vi "Replace Child.vi"(7 "Children In Place? (F)":bool, 8 "error in (no error)":errorcluster, 9 "New Node":refnum<data-value>, 10 "Old Node":refnum<data-value>, 11 "NodeRef In":refnum<data-value>) -> (0 "error out":errorcluster, 3 "NodeRef":refnum<data-value>)   [LabVIEW 2020, in "PicoG-ParserLexer.lvlib" / "Node.lvclass"]
uses:
  Node.lvclass
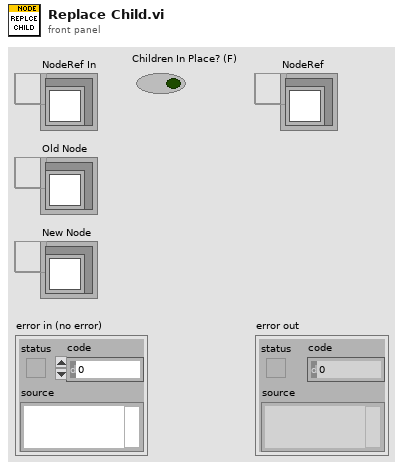
[diagram p1: front panel]
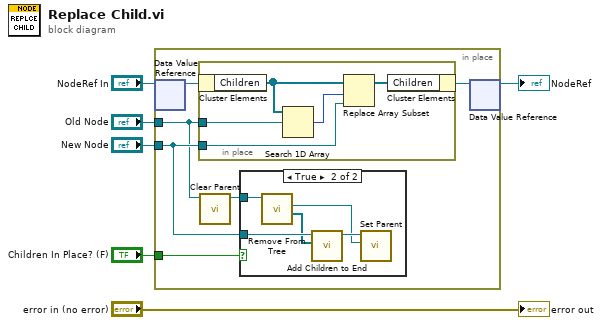
[diagram p0: block diagram]
diagram:
  n1 = in-place {
    in-place-border: "Old Node" -> [w7]
    in-place-border: "New Node" -> [w9]
    in-place-border: "Children In Place? (F)" -> [w10]
    n2 = in-place-dvr #1("NodeRef In") -> (w12:refnum<class "Node.lvclass">)  [unwired: 1 out]
    n3 = in-place {
      in-place-border: w7 -> [w22]
      in-place-border: w9 -> [w19]
      n4 = in-place-cluster #2(w12) -> ("Children"=w21:refnum<data-value>[])
      n5 = Search 1D Array(1D array=w21, element=w22) -> (index of element=w20:i32)  [unwired: 1 in]
      n6 = Replace Array Subset(array=w21, new element=w19, index=w20) -> (w18:refnum<data-value>[])
      n7 = in-place-cluster #2("Children"=w18) -> (w11:refnum<class "Node.lvclass">)
    }
    n8 = call "Clear Parent.vi"("NodeRef In"=w7) -> ("NodeRef"=w8:refnum<data-value>)  [unwired: 9 in, 1 out]
    n9 = case shown="True" w10 {
      tunnel: w8 -> [_ w17]
      tunnel: w9 -> [_ w16]
      frame False {
        # "Children stay with removed node."
      }
      frame True {
        n10 = call "Remove From Tree.vi"("NodeRef In"=w17) -> ("Children"=w15:refnum<data-value>[], "Parent"=w13:refnum<data-value>)  [unwired: 7 in, 2 out]
        n11 = call "Add Children to End.vi"("Children"=w15, "NodeRef In"=w16) -> ("NodeRef"=w14:refnum<data-value>)  [unwired: 8 in, 1 out]
        n12 = call "Set Parent.vi"("Parent"=w13, "NodeRef In"=w14) -> ()  [unwired: 8 in, 2 out]
      }
    }
    n13 = in-place-dvr #1(w11) -> (→"NodeRef":refnum<data-value>)  [unwired: 1 out]
  }
  "error out" <- "error in (no error)"
